vi "rs3 delete device list.vi"(8 "error in (no error)":errorcluster, 11 "device list":u64) -> (0 "error out":errorcluster)   [LabVIEW 2023]
doc: "Delete the device list after all devices have been deleted."
panel:
  # "RS3 Delete Device List"
  # "(C) Intel Corp. 2017,  AGJ"
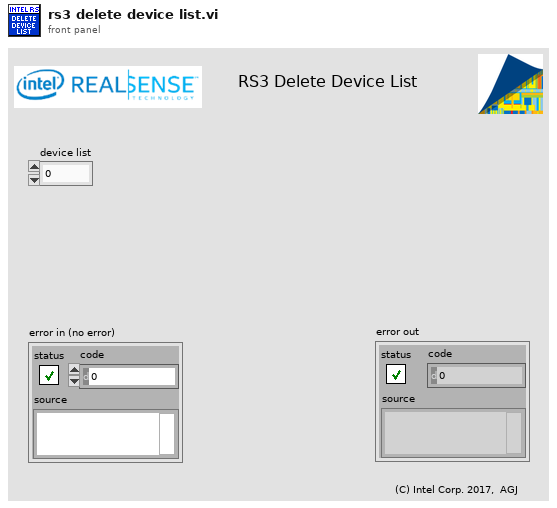
[diagram p1: front panel]
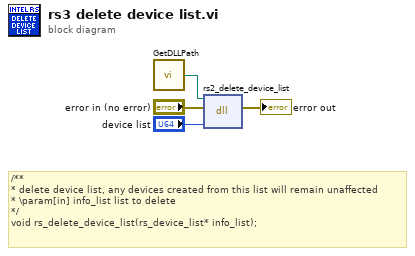
[diagram p0: block diagram]
diagram:
  # "/**\n* delete device list, any devices created from this list will remain unaffected\n* \\param[in] info_list list to delete\n*/\nvoid rs_delete_device_list(rs_device_list* info_list);"
  n1 = call "GetDLLPath.vi"() -> ("DLL Path"=w1:path)
  n2 = dll-call lib="C:/STEAMSyndicate/RealSenseWrappers/VI Wrappers (add ons) Public/RealSense/realsense2.dll" fn="rs2_delete_device_list"(path in=w1, error in="error in (no error)", "device list"="device list") -> (error out=→"error out":errorcluster)  [unwired: 3 in, 1 out]
